vi "Init.vi"(8 "error in":errorcluster, 10 "Object Dictionary":refnum<class "Object Dictionary.lvclass">, 11 "Sorted Object Dictionary in":refnum<class "Sorted Object Dictionary.lvclass">) -> (0 "error out":errorcluster, 3 "Sorted Object Dictionary out":refnum<class "Sorted Object Dictionary.lvclass">)   [LabVIEW 2024, in "EDS.lvlib" / "Sorted Object Dictionary.lvclass"]
uses:
  Sorted Object Dictionary.lvclass
  Sorted Object Dictionary.lvclass/Sorted Object Dictionary.ctl
  Object Dictionary/Object Dictionary.lvclass
  OD Section/OD Section.lvclass
  OD Entry/OD Entry.lvclass
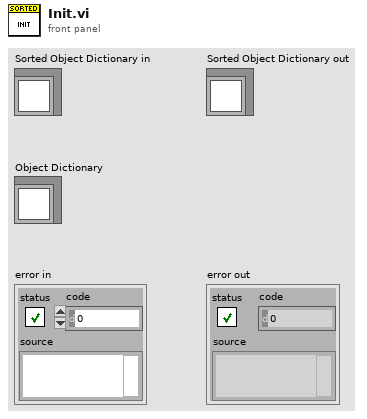
[diagram p1: front panel]
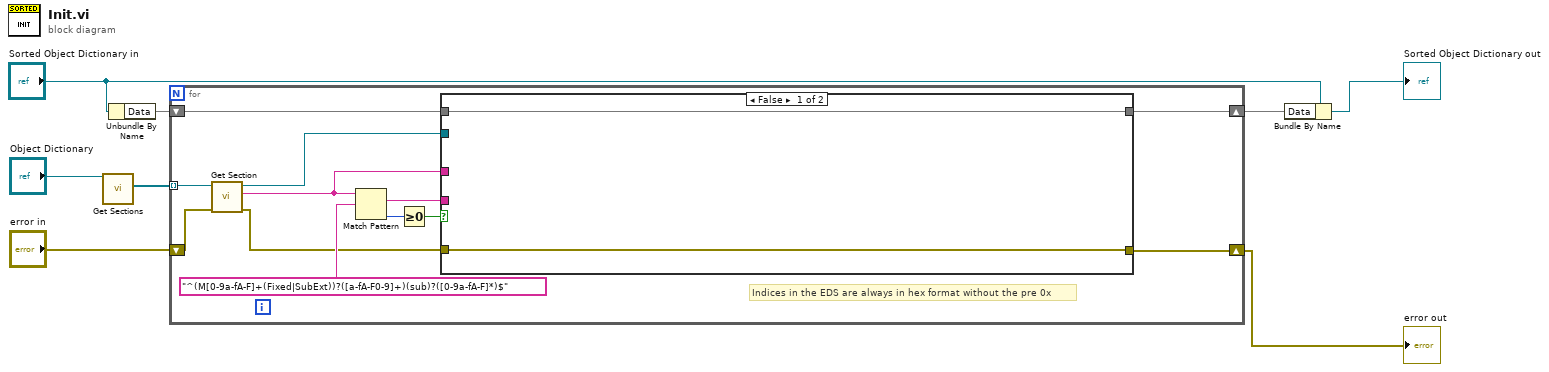
[diagram p0: block diagram]
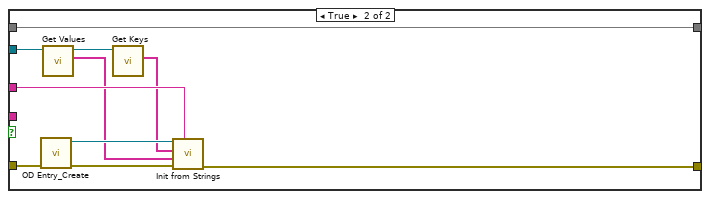
[diagram p2: hidden frame]
diagram:
  n1 = call "Get Sections.vi"("Object Dictionary in"="Object Dictionary") -> ("OD Sections"=w7:refnum<class "OD Section.lvclass">[])  [unwired: 9 in, 1 out]
  n2 = Unbundle By Name("Sorted Object Dictionary in") -> ("Data"=w6:map{u16, refnum<class "OD Entry.lvclass">})
  n3 = for {
    tunnel: w7 -> [w19] mode=indexing
    shift-right: [w10] -> w3
    shift-left: w6 -> [w11]
    shift-right: [w9] -> w1
    shift-left: "error in" -> [w14]
    # "Indices in the EDS are always in hex format without the pre 0x"
    n4 = call "Get Section.vi"("error in"=w14, "Object Entry in"=w19) -> ("error out"=w13:errorcluster, "Section"=w15:string, "Object Entry out"=w12:refnum<class "OD Section.lvclass">)  [unwired: 7 in]
    n5 = Match Pattern(string=w15, regular expression="^(M[0-9a-fA-F]+(Fixed|SubExt))?([a-fA-F0-9]+)(sub)?([0-9a-fA-F]*)$") -> (match substring=w16:string, offset past match=w18:i32)  [unwired: 1 in, 2 out]
    n6 = Greater Or Equal To 0?(x=w18) -> (x >= 0?=w17:bool)
    n7 = case shown="False" w17 {
      tunnel: w16 -> [_ _]
      tunnel: w15 -> [_ w29]
      tunnel: w13 -> [w22 w32]
      tunnel: w12 -> [_ w26]
      tunnel: w11 -> [w21 w24]
      tunnel: [w21 w24] -> w10
      tunnel: [w22 w23] -> w9
      frame False {
      }
      frame True {
        n8 = call "OD Entry_Create.vi"("Error In"=w32) -> ("Error Out"=w31:errorcluster, "reference out"=w30:refnum<class "OD Entry.lvclass">)  [unwired: 9 in]
        n9 = call "Get Values.vi"("Object Entry in"=w26) -> ("Values"=w27:string[], "Object Entry out"=w25:refnum<class "OD Section.lvclass">)  [unwired: 8 in, 1 out]
        n10 = call "Get Keys.vi"("Object Entry in"=w25) -> ("Keys"=w28:string[])  [unwired: 8 in, 2 out]
        n11 = call "Init from Strings.vi"("Index"=w29, "Error In"=w31, "Values"=w27, "Keys"=w28, "reference in"=w30) -> ("Error Out"=w23:errorcluster)  [unwired: 5 in, 1 out]
      }
    }
  }
  "error out" <- w1
  n12 = Bundle By Name(cluster="Sorted Object Dictionary in", "Data"=w3) -> (→"Sorted Object Dictionary out":refnum<class "Sorted Object Dictionary.lvclass">)
